vi "Update Cursor Indicator.vi"(8 "error in (no error)":errorcluster, 9 "Cursor Info":T1, 10 "Time/Div":string, 11 "Program Data":T2={"Measurements"={"Channel 0"="Channel 0", "RMS 0"="RMS:", "Vp-p 0"="Vp-p:", "Freq 0"="Freq:", "Channel 1"="Channel 1", "RMS 1"="RMS:", "Vp-p 1"="Vp-p:", "Freq 1"="Freq:", "Cursors"="Channel 0", "C1"="Channel 0", "C2"="Channel 0", "dT"="Channel 0"}, "C1"={"Name"="", "X"=0.0, "Y"=0.0}, "C2"={"Name"="", "X"=0.0, "Y"=0.0}, "Com"={"Connection Info"={"connection ID"=refnum, "meta data"=[]}, "Connected?"=FALSE, "IP"=""}, "Continuous?"=FALSE, "Scope Data"={"AI0"=[], "AI1"=[]}, "Wave Parameters"={"Frequency (Hz)"=5.0, "Phase offset (deg)"=0.0, "Vpeak (V)"=5.0, "Offset (V)"=0.0, "Waveform"=enum."Sine", "Channel"=enum."CH0"}, "Acquire?"=FALSE, "Measure Ref"=refnum, "CH0"={"Channel"=enum."AI 0", "Enable"=FALSE, "Volts/Div"=0, "Vertical Position (Div)"=0.0}, "CH1"={"Channel"=enum."AI 0", "Enable"=FALSE, "Volts/Div"=0, "Vertical Position (Div)"=0.0}, "CH0 Params"={"V/Div"=0.0, "Units"=""}, "CH1 Params"={"V/Div"=0.0, "Units"=""}, "Time"={"Time/Div"=0.0}, "dT"=0.0, "FGen"={"Offset (V)"=0.0, "Enable Sweep"=FALSE, "Start Frequency (Hz)"=0.0, "Stop Frequency (Hz)"=0.0, "Step (Hz)"=0.0, "Step Interval (ms)"=0.0, "Current Freq (Hz)"=0.0, "Run"=FALSE}} {"Time"."Time/Div" min=0.0 max=16.0 step=1.0 scale=0.0..12.0; "CH1"."Vertical Position (Div)" min=-5.0 max=5.0 step=0.1 scale=-5.0..5.0; "CH1"."Volts/Div" min=0 max=8 step=1 scale=0.0..8.0; "CH0"."Vertical Position (Div)" min=-5.0 max=5.0 step=0.1 scale=-5.0..5.0; "CH0"."Volts/Div" min=0 max=8 step=1 scale=0.0..8.0; "Wave Parameters"."Phase offset (deg)" format="%#_6p"; "Wave Parameters"."Frequency (Hz)" format="%#_6p"}) -> (0 "error out":errorcluster, 3 "Program Data Out":T2={"Measurements"={"Channel 0"="Channel 0", "RMS 0"="RMS:", "Vp-p 0"="Vp-p:", "Freq 0"="Freq:", "Channel 1"="Channel 1", "RMS 1"="RMS:", "Vp-p 1"="Vp-p:", "Freq 1"="Freq:", "Cursors"="Channel 0", "C1"="Channel 0", "C2"="Channel 0", "dT"="Channel 0"}, "C1"={"Name"="", "X"=0.0, "Y"=0.0}, "C2"={"Name"="", "X"=0.0, "Y"=0.0}, "Com"={"Connection Info"={"connection ID"=refnum, "meta data"=[]}, "Connected?"=FALSE, "IP"=""}, "Continuous?"=FALSE, "Scope Data"={"AI0"=[], "AI1"=[]}, "Wave Parameters"={"Frequency (Hz)"=5.0, "Phase offset (deg)"=0.0, "Vpeak (V)"=5.0, "Offset (V)"=0.0, "Waveform"=enum."Sine", "Channel"=enum."CH0"}, "Acquire?"=FALSE, "Measure Ref"=refnum, "CH0"={"Channel"=enum."AI 0", "Enable"=FALSE, "Volts/Div"=0, "Vertical Position (Div)"=0.0}, "CH1"={"Channel"=enum."AI 0", "Enable"=FALSE, "Volts/Div"=0, "Vertical Position (Div)"=0.0}, "CH0 Params"={"V/Div"=0.0, "Units"=""}, "CH1 Params"={"V/Div"=0.0, "Units"=""}, "Time"={"Time/Div"=0.0}, "dT"=0.0, "FGen"={"Offset (V)"=0.0, "Enable Sweep"=FALSE, "Start Frequency (Hz)"=0.0, "Stop Frequency (Hz)"=0.0, "Step (Hz)"=0.0, "Step Interval (ms)"=0.0, "Current Freq (Hz)"=0.0, "Run"=FALSE}} {"Time"."Time/Div" min=0.0 max=16.0 step=1.0 scale=0.0..12.0; "CH1"."Vertical Position (Div)" min=-5.0 max=5.0 step=0.1 scale=-5.0..5.0; "CH1"."Volts/Div" min=0 max=8 step=1 scale=0.0..8.0; "CH0"."Vertical Position (Div)" min=-5.0 max=5.0 step=0.1 scale=-5.0..5.0; "CH0"."Volts/Div" min=0 max=8 step=1 scale=0.0..8.0; "Wave Parameters"."Phase offset (deg)" format="%#_6p"; "Wave Parameters"."Frequency (Hz)" format="%#_6p"})   [LabVIEW 2018]
uses:
  Controls/Program Data.ctl
  Controls/Measurements.ctl
  Controls/Channel Measurement String Control.ctl
  Controls/Cursor Info.ctl
  Controls/Communication Cluster.ctl
  <vilib>/NI/STM/TCP/TCP Connection Info.ctl
  <vilib>/NI/STM/SubVIs/MetaDataElement.ctl
  Communication/Scope Data.ctl
  Program Files (x86)/National Instruments/LabVIEW 2018/ProjectTemplates/Source/myRIO/Oscilloscope/myRIO v1.1/Real-Time/Controls/Wave Parameters.ctl
  Program Files (x86)/National Instruments/LabVIEW 2018/ProjectTemplates/Source/myRIO/Oscilloscope/myRIO v1.1/Real-Time/Controls/Waveform Enum.ctl
  Program Files (x86)/National Instruments/LabVIEW 2018/ProjectTemplates/Source/myRIO/Oscilloscope/myRIO v1.1/Real-Time/Controls/Channel Selector.ctl
  Controls/Channel Settings.ctl
  Controls/Analog Input Selector.ctl
  Controls/Knob.ctl
  Controls/Vertical Position.ctl
  Controls/Channel Parameters.ctl
  Controls/Time Selector.ctl
  Controls/Time Knob.ctl
  Controls/FGen Desktop Configuration.ctl
  <vilib>/NI/STM/NI STM.lvlib
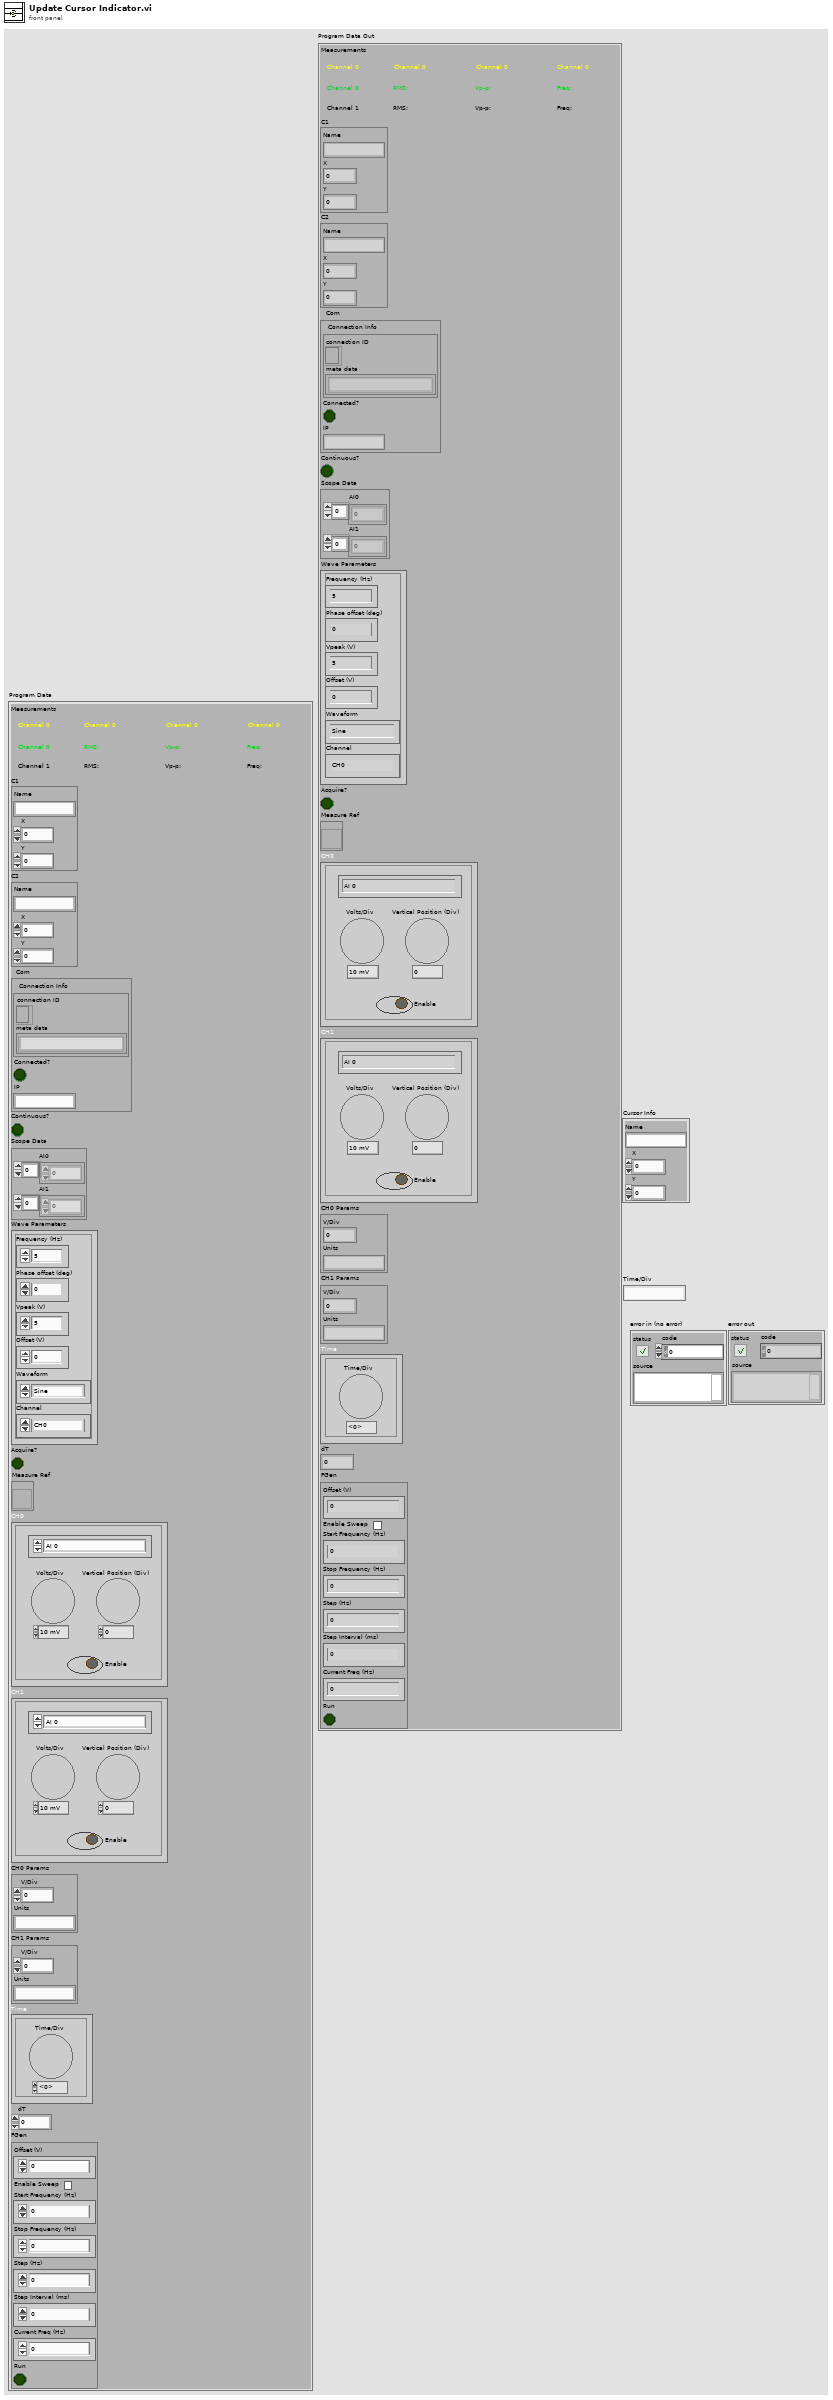
[diagram p1: front panel]
types:
  T1 = typedef "Cursor Info.ctl" = cluster{"Name":string, "X":dbl, "Y":dbl}
  T2 = typedef "Program Data.ctl" = cluster{"Measurements":T3, "C1":T1, "C2":T1, "Com":T5, "Continuous?":bool, "Scope Data":T8, "Wave Parameters":T9, "Acquire?":bool, "Measure Ref":refnum<vi>, "CH0":T12, "CH1":T12, "CH0 Params":T16, "CH1 Params":T16, "Time":T17, "dT":dbl, "FGen":T19}
  T3 = typedef "Measurements.ctl" = cluster{"Channel 0":T4, "RMS 0":T4, "Vp-p 0":T4, "Freq 0":T4, "Channel 1":T4, "RMS 1":T4, "Vp-p 1":T4, "Freq 1":T4, "Cursors":T4, "C1":T4, "C2":T4, "dT":T4}
  T4 = typedef "Channel Measurement String Control.ctl" = string
  T5 = typedef "Communication Cluster.ctl" = cluster{"Connection Info":T6, "Connected?":bool, "IP":string}
  T6 = typedef "NI STM.lvlib/TCP Connection Info.ctl" = cluster{"connection ID":refnum<k5>, "meta data":T7[]}
  T7 = typedef "NI STM.lvlib/MetaDataElement.ctl" = string
  T8 = typedef "Scope Data.ctl" = cluster{"AI0":dbl[], "AI1":dbl[]}
  T9 = typedef "Wave Parameters.ctl" = cluster{"Frequency (Hz)":dbl, "Phase offset (deg)":dbl, "Vpeak (V)":dbl, "Offset (V)":dbl, "Waveform":T10, "Channel":T11}
  T10 = typedef "Waveform Enum.ctl" = enum16{"Sine", "Square"}
  T11 = typedef "Channel Selector.ctl" = enum16{"CH0", "CH1"}
  T12 = typedef "Channel Settings.ctl" = cluster{"Channel":T13, "Enable":bool, "Volts/Div":T14, "Vertical Position (Div)":T15}
  T13 = typedef "Analog Input Selector.ctl" = enum16{"AI 0", "AI 1"}
  T14 = typedef "Knob.ctl" = i32
  T15 = typedef "Vertical Position.ctl" = dbl
  T16 = typedef "Channel Parameters.ctl" = cluster{"V/Div":dbl, "Units":string}
  T17 = typedef "Time Selector.ctl" = cluster{"Time/Div":T18}
  T18 = typedef "Time Knob.ctl" = dbl
  T19 = typedef "FGen Desktop Configuration.ctl" = cluster{"Offset (V)":dbl, "Enable Sweep":bool, "Start Frequency (Hz)":dbl, "Stop Frequency (Hz)":dbl, "Step (Hz)":dbl, "Step Interval (ms)":dbl, "Current Freq (Hz)":dbl, "Run":bool}
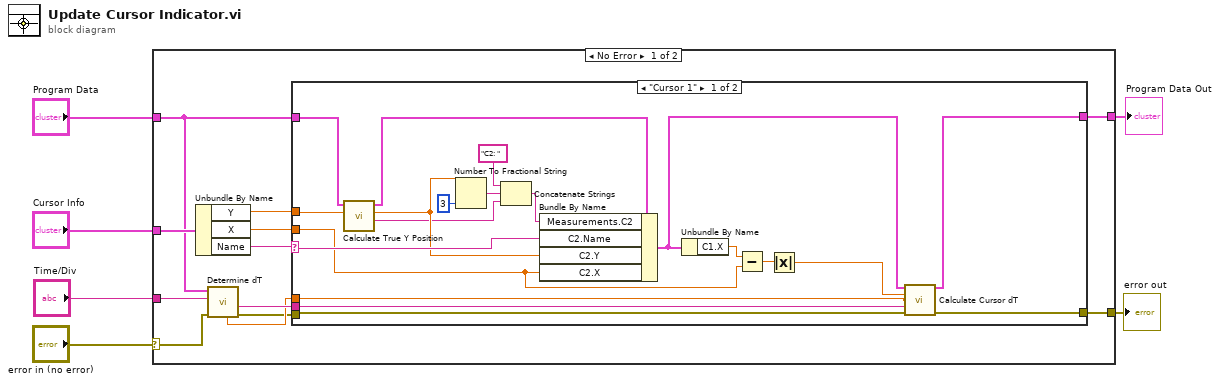
[diagram p0: block diagram]
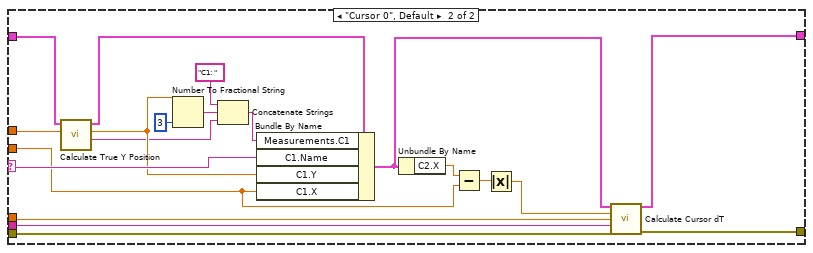
[diagram p2: hidden frame]
diagram:
  n1 = case shown="No Error" "error in (no error)" {
    selector: "error in (no error)" -> [w11 w59]
    tunnel: "Cursor Info" -> [w18 _]
    tunnel: "Program Data" -> [w12 w60]
    tunnel: [w16 w60] -> w4
    tunnel: "Time/Div" -> [w13 _]
    tunnel: [w7 w59] -> w1
    frame No Error {
      n2 = Unbundle By Name(w18) -> ("Y"=w17:dbl, "X"=w15:dbl, "Name"=w14:string)
      n3 = call "Determine dT.vi"("error in (no error)"=w11, "Time/Div"=w13, "Program Data"=w12) -> ("error out"=w8:errorcluster, "Units"=w10:string, "Time"=w9:dbl)  [unwired: 4 in, 2 out]
      n4 = case shown="\"Cursor 1\"" w14 {
        selector: w14 -> [w34 w54]
        tunnel: w12 -> [w29 w47]
        tunnel: w17 -> [w30 w48]
        tunnel: [w19 w49] -> w16
        tunnel: w15 -> [w32 w52]
        tunnel: w9 -> [w22 w42]
        tunnel: w10 -> [w23 w41]
        tunnel: w8 -> [w24 w40]
        tunnel: [w25 w39] -> w7
        frame "Cursor 1" {
          n5 = call "Calculate True Y Position.vi"("Y Position"=w30, "Program Data"=w29) -> ("Units"=w26:string, "True Y Position"=w27:T15, "Program Data Out"=w28:T2)  [unwired: 6 in, 1 out]
          n6 = Number To Fractional String(number=w27, precision (6)=i16 3) -> (F-format string=w38:string)  [unwired: 2 in]
          n7 = Concatenate Strings("C2: " ("string"), w38, w26) -> (w36:string)
          n8 = Bundle By Name(cluster=w28, "Measurements.C2"=w36, "C2.Name"=w34, "C2.Y"=w27, "C2.X"=w32) -> (w20:T2)
          n9 = Unbundle By Name(w20) -> ("C1.X"=w33:dbl)
          n10 = Subtract(x=w33, y=w32) -> (x-y=w31:dbl)
          n11 = Absolute Value(x=w31) -> (abs(x)=w21:dbl)
          n12 = call "Calculate Cursor dT.vi"("Program Data In"=w20, "Cursor X Difference"=w21, "Time/pt"=w22, "Units"=w23, "error in (no error)"=w24) -> ("Program Data Out"=w19:T2, "error out"=w25:errorcluster)  [unwired: 9 in]
        }
        frame "Cursor 0", Default {
          n13 = call "Calculate True Y Position.vi"("Y Position"=w48, "Program Data"=w47) -> ("Units"=w44:string, "True Y Position"=w45:T15, "Program Data Out"=w46:T2)  [unwired: 6 in, 1 out]
          n14 = Number To Fractional String(number=w45, precision (6)=i16 3) -> (F-format string=w58:string)  [unwired: 2 in]
          n15 = Concatenate Strings("C1: " ("string"), w58, w44) -> (w56:string)
          n16 = Bundle By Name(cluster=w46, "Measurements.C1"=w56, "C1.Name"=w54, "C1.Y"=w45, "C1.X"=w52) -> (w50:T2)
          n17 = Unbundle By Name(w50) -> ("C2.X"=w53:dbl)
          n18 = Subtract(x=w53, y=w52) -> (x-y=w51:dbl)
          n19 = Absolute Value(x=w51) -> (abs(x)=w43:dbl)
          n20 = call "Calculate Cursor dT.vi"("Program Data In"=w50, "Cursor X Difference"=w43, "Time/pt"=w42, "Units"=w41, "error in (no error)"=w40) -> ("Program Data Out"=w49:T2, "error out"=w39:errorcluster)  [unwired: 9 in]
        }
      }
    }
    frame Error {
    }
  }
  "Program Data Out" <- w4
  "error out" <- w1
